vi "VariableGet.vi"(8 "error in (no error)":errorcluster, 10 "VariableName":string, 11 "VariableManagerRef in":refnum<vi>) -> (0 "error out":errorcluster, 2 "Variable":refnum<class "Variable.lvclass">, 3 "VariableManagerRef out":refnum<vi>)   [LabVIEW 2013, in "VariableManagerAPI.lvlib"]
doc: "Return variable definition of VariableName.\n\nAn error is thrown if a VariableName does not exist."
uses:
  VariableManagerAPI.lvlib
  VariableManager/VariableManager.lvclass
  Variable/Variable.lvclass
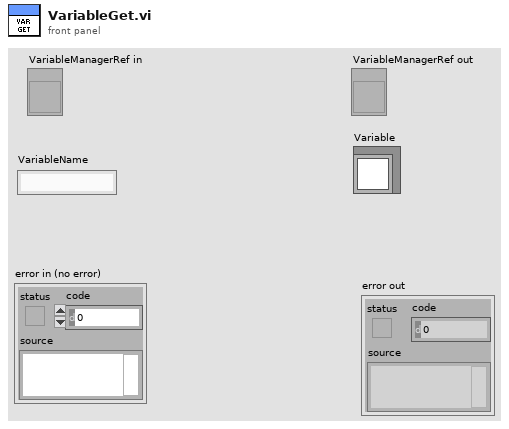
[diagram p1: front panel]
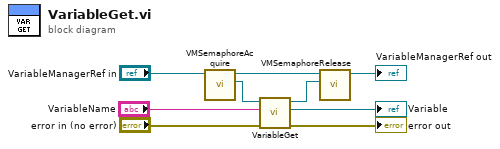
[diagram p0: block diagram]
diagram:
  n1 = call "VMSemaphoreAcquire.vi"("VariableManagerRef in"="VariableManagerRef in") -> ("VariableManager"=w6:refnum<class "VariableManager.lvclass">, "VariableManagerRef out"=w8:refnum<vi>)  [unwired: 7 in, 2 out]
  n2 = call-dynamic "VariableGet.vi"("error in (no error)"="error in (no error)", "VariableName"="VariableName", "VariableManager in"=w6) -> ("error out"=→"error out":errorcluster, "Variable"=→"Variable":refnum<class "Variable.lvclass">, "VariableManager out"=w5:refnum<class "VariableManager.lvclass">)  [unwired: 6 in]
  n3 = call "VMSemaphoreRelease.vi"("VariableManager"=w5, "VariableManagerRef in"=w8) -> ("VariableManagerRef out"=→"VariableManagerRef out":refnum<vi>)  [unwired: 8 in, 1 out]
